vi "Sawtooth Wave PtByPt.vi"(1 "time":dbl format="%0.2f", 2 "phase":dbl format="%0.2f", 3 "frequency":dbl=1.0 format="%0.2f", 4 "amplitude":dbl=1.0 format="%0.2f") -> (0 "sawtooth wave":dbl format="%0.2f")   [LabVIEW 2020, in "NI_PtbyPt.lvlib"]
doc: "Generates a sawtooth wave point by point."
uses:
  <vilib>/ptbypt/NI_PtbyPt.lvlib
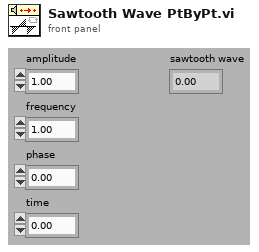
[diagram p1: front panel]
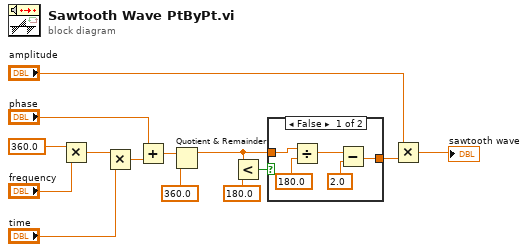
[diagram p0: block diagram]
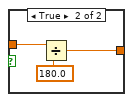
[diagram p2: hidden frame]
diagram:
  n1 = Multiply(x=360.0, y="frequency") -> (x*y=w13:dbl)
  n2 = Multiply(x=w13, y="time") -> (x*y=w8:dbl)
  n3 = Add(x="phase", y=w8) -> (x+y=w7:dbl)
  n4 = Quotient & Remainder(x=w7, y=360.0) -> (x-y*floor(x/y)=w3:dbl)  [unwired: 1 out]
  n5 = Less?(x=w3, y=180.0) -> (x < y?=w4:bool)
  n6 = case shown="False" w4 {
    tunnel: w3 -> [w19 w21]
    tunnel: [w15 w20] -> w2
    frame False {
      n7 = Divide(x=w19, y=180.0) -> (x/y=w17:dbl)
      n8 = Subtract(x=w17, y=2.0) -> (x-y=w15:dbl)
    }
    frame True {
      n9 = Divide(x=w21, y=180.0) -> (x/y=w20:dbl)
    }
  }
  n10 = Multiply(x="amplitude", y=w2) -> (x*y=→"sawtooth wave":dbl)
